vi "Set Defaults.vi"(11 "Entity in":refnum<class "Entity.lvclass">) -> (3 "Entity out":refnum<class "Entity.lvclass">)   [LabVIEW 2020, in "Conditu2.lvlib" / "Entity.lvclass"]
uses:
  Entity.lvclass
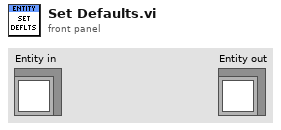
[diagram p1: front panel]
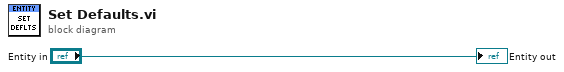
[diagram p0: block diagram]
diagram:
  "Entity out" <- "Entity in"
